vi "create.vi"(0 "MTILCFactory in":refnum<class "MTILCFactory.lvclass">, 5 "MTSettings":T3, 7 "ILCTimings":T1, 9 "MTTimings":T2, 11 "error in (no error)":errorcluster) -> (4 "MTILCFactory out":refnum<class "MTILCFactory.lvclass">, 6 "MTILC":refnum<class "MTILC.lvclass">, 15 "error out":errorcluster)   [LabVIEW 2016, in "RTMTILC.lvlib" / "MTILCFactory.lvclass"]
uses:
  MTILCFactory.lvclass
  DataTypes/MTSettings.ctl
  Common_RT_ILC/DataTypes/ILCSettings.ctl
  MTILC/MTILC.lvclass
  D:/Code/Common_RT_ILC/ILC/ILC.lvclass
  DataTypes/MTTimings.ctl
  Common_RT_ILC/DataTypes/ILCTimings.ctl
  Common_RT_ILC/ILCFactory/ILCFactory.lvclass
  DataTypes/MTData.ctl
  DataTypes/MTConstants.ctl
  DataTypes/MTTelemetry.ctl
  DataTypes/MTResponses.ctl
  Common_RT_Modbus/DataTypes/ExceptionCodes.ctl
  MTILC/MTILC.lvclass/MTILC.ctl
  RTMTILC.lvlib
  Common_RT_Modbus/RTModbus.lvlib
  Common_RT_ILC/RTILC.lvlib
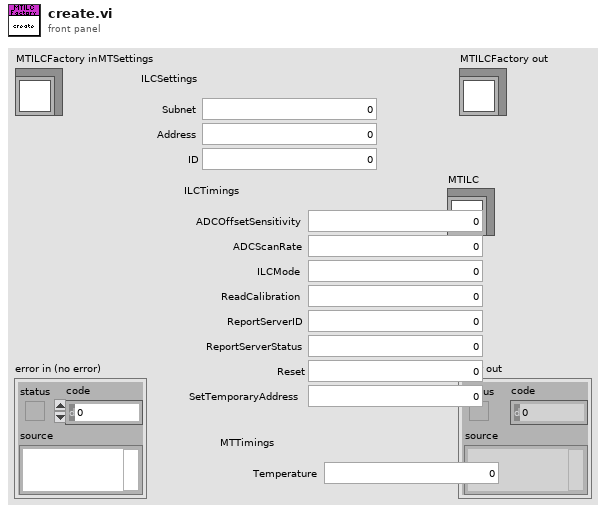
[diagram p1: front panel]
types:
  T1 = typedef "RTILC.lvlib/ILCTimings.ctl" = cluster{"ADCOffsetSensitivity":u32, "ADCScanRate":u32, "ILCMode":u32, "ReadCalibration":u32, "ReportServerID":u32, "ReportServerStatus":u32, "Reset":u32, "SetTemporaryAddress":u32}
  T2 = typedef "RTMTILC.lvlib/MTTimings.ctl" = cluster{"Temperature":u32}
  T3 = typedef "RTMTILC.lvlib/MTSettings.ctl" = cluster{"ILCSettings":T4, "ID":i16}
  T4 = typedef "RTILC.lvlib/ILCSettings.ctl" = cluster{"Subnet":u8, "Address":u8}
  T5 = typedef "RTMTILC.lvlib/MTData.ctl" = cluster{"Constants":T6, "Telemetry":T7, "Responses":T8, "Timings":T2}
  T6 = typedef "RTMTILC.lvlib/MTConstants.ctl" = cluster{"ID":i16}
  T7 = typedef "RTMTILC.lvlib/MTTelemetry.ctl" = cluster{"Temperature":sgl[]}
  T8 = typedef "RTMTILC.lvlib/MTResponses.ctl" = cluster{"Temperature":T9}
  T9 = typedef "RTModbus.lvlib/ExceptionCodes.ctl" = u16
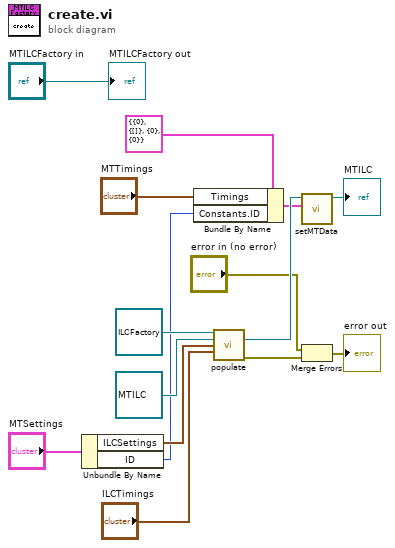
[diagram p0: block diagram]
diagram:
  n1 = Unbundle By Name("MTSettings") -> ("ILCSettings"=w14:T4, "ID"=w9:i16)
  n2 = Bundle By Name(cluster=T5 {"Constants"={"ID"=0}, "Telemetry"={"Temperature"=[]}, "Responses"={"Temperature"=0}, "Timings"={"Temperature"=0}} ("MTData"), "Timings"="MTTimings", "Constants.ID"=w9) -> (w8:T5)
  n3 = call "populate.vi"("ILCFactory in"=refnum<class "ILCFactory.lvclass"> refnum ("RTILC.lvlib:ILCFactory.lvclass"), "ILC in"=refnum<class "MTILC.lvclass"> refnum ("RTMTILC.lvlib:MTILC.lvclass"), "Settings"=w14, "Timings"="ILCTimings") -> ("ILC out"=w11:refnum<class "MTILC.lvclass">, "error out"=w6:errorcluster)  [unwired: 9 in, 1 out]
  n4 = call "setMTData.vi"("MTData"=w8, "MTILC in"=w11) -> ("MTILC out"=→"MTILC":refnum<class "MTILC.lvclass">)  [unwired: 9 in]
  n5 = Merge Errors("error in (no error)", w6) -> (→"error out":errorcluster)
  "MTILCFactory out" <- "MTILCFactory in"
